vi "Hardware_auto_params_set_test.vi"() -> ()   [LabVIEW 2018]
uses:
  <vilib>/nisyscfg/Close (Resources).vi
  <vilib>/nisyscfg/Close (System).vi
  <vilib>/nisyscfg/nisyscfg.lvlib
  <resource>/objmgr/nicontrollersysapi.rc
  <resource>/objmgr/nisysapi.rc
panel:
  out "Port binding":string[](array[string])
  out "error out":errorcluster
  out "Alias":string[](array[string])
  out "Resource":string[](array[string])
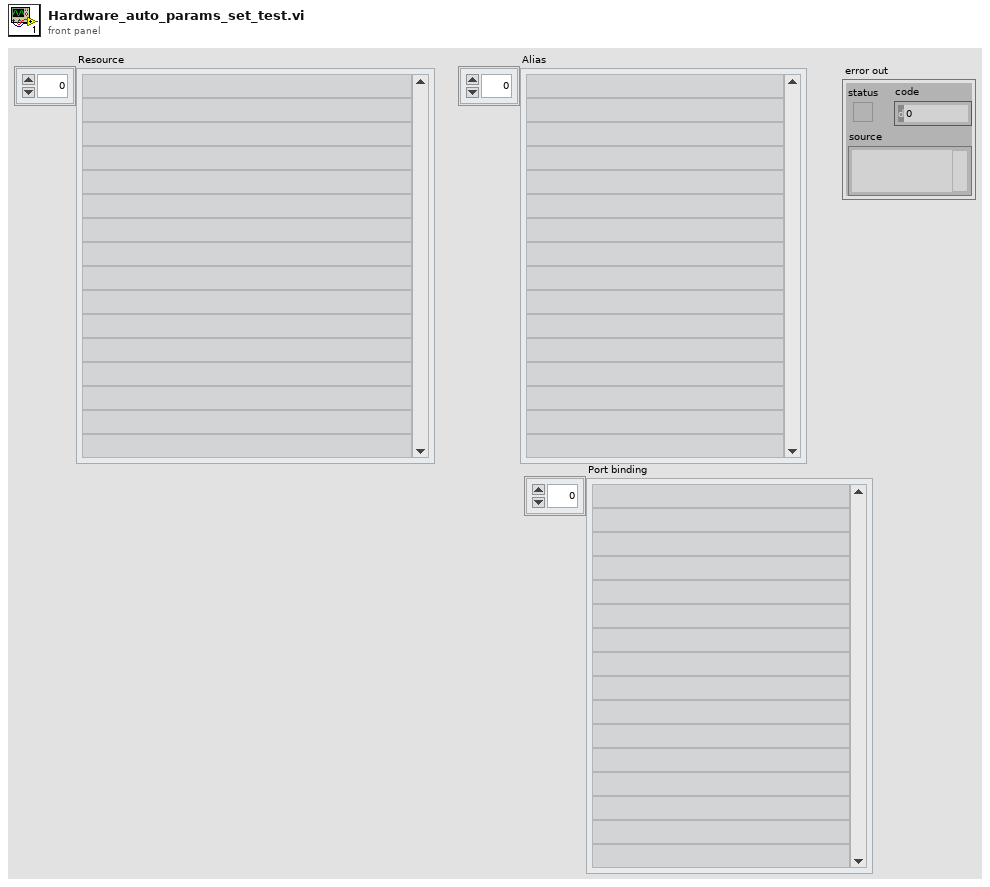
[diagram p1: front panel]
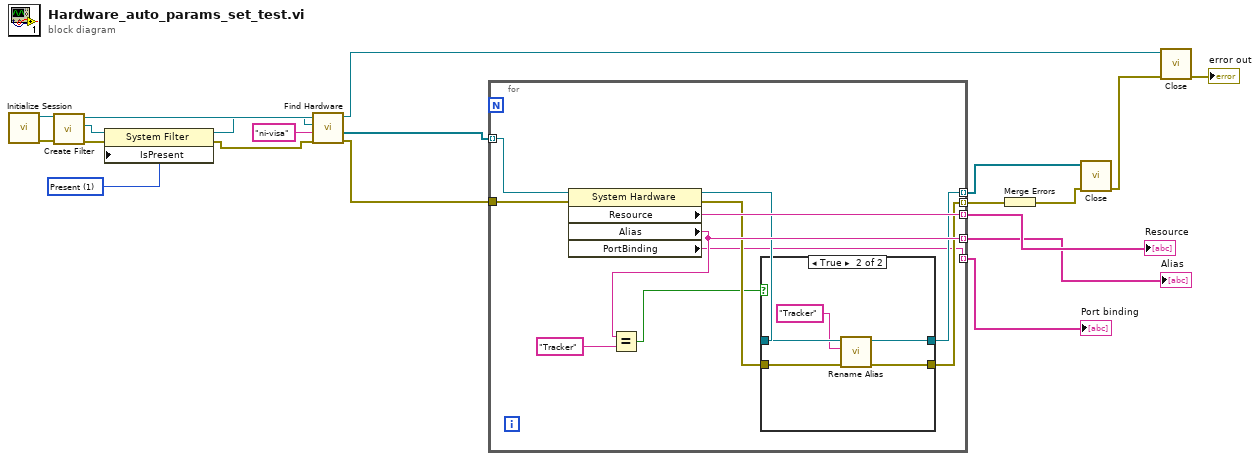
[diagram p0: block diagram]
diagram:
  w8 = 1 items=["Initializing"=-2, "Unknown"=-1, "Not Present"=0, "Present"=1] ("Devices & Chassis:Is Present")
  n1 = call <vilib>:"Initialize Session.vi"() -> ("error out"=w6:errorcluster, "Session out"=w7:refnum<k21>)  [unwired: 10 in]
  n2 = call <vilib>:"Create Filter.vi"("error in (no error)"=w6, "Session in"=w7) -> ("error out"=w10:errorcluster, "Filter out"=w9:refnum<k20>, "Session out"=w5:refnum<k21>)  [unwired: 7 in]
  n3 = property class="System Filter"(reference=w9, error in=w10, "IsPresent"=w8) -> (reference out=w3:refnum<k20>, error out=w4:errorcluster)
  n4 = call <vilib>:"Find Hardware.vi"("error in (no error)"=w4, "Experts"="ni-visa", "Filter in"=w3, "Session in"=w5) -> ("error out"=w17:errorcluster, "Resources out"=w20:refnum<k20>[], "Session out"=w14:refnum<k21>)  [unwired: 4 in, 1 out]
  n5 = for {
    tunnel: w20 -> [w31] mode=indexing
    tunnel: [w30] -> w19 mode=indexing
    tunnel: [w23] -> w18 mode=indexing
    tunnel: w17 -> [w29]
    tunnel: [w24] -> w16 mode=indexing
    tunnel: [w28] -> w12 mode=indexing
    tunnel: [w21] -> w1 mode=indexing
    n6 = property class="System Hardware"(reference=w31, error in=w29) -> (reference out=w26:refnum<k20>, error out=w25:errorcluster, "Resource"=w30:string, "Alias"=w28:string, "PortBinding"=w21:string)
    n7 = Equal?(x=w28, y="Tracker") -> (x = y?=w22:bool)
    n8 = case shown="True" w22 {
      tunnel: w26 -> [w33 w38]
      tunnel: w25 -> [w32 w37]
      tunnel: [w32 w36] -> w24
      tunnel: [w33 w35] -> w23
      frame False {
      }
      frame True {
        n9 = call <vilib>:"Rename Alias.vi"("error in (no error)"=w37, "New Name"="Tracker", "Resource in"=w38) -> ("error out"=w36:errorcluster, "Resource out"=w35:refnum<k20>)  [unwired: 5 in, 2 out]
      }
    }
  }
  "Resource" <- w19
  "Alias" <- w12
  "Port binding" <- w1
  n10 = Merge Errors(w16) -> (w15:errorcluster)
  n11 = call-poly <vilib>:"Close.vi"("error in (no error)"=w15, "Resources in"=w18) -> ("error out"=w13:errorcluster)  [unwired: 9 in]
  n12 = call-poly <vilib>:"Close.vi"("error in (no error)"=w13, "Session in"=w14) -> ("error out"=→"error out":errorcluster)  [unwired: 9 in]
